vi "RT_MAIN.vi"() -> ()   [LabVIEW 2019]
uses:
  <vilib>/Platform/TimedLoop/XDataNode/timing_clust.ctl
  <vilib>/Platform/TimedLoop/XDataNode/nitl_modes.ctl
  <vilib>/Platform/TimedLoop/XDataNode/wakeup.ctl
  <vilib>/FPGAPlugInAG/cRIO-9040/niLvFpga_Open_cRIO-9040.vi
  <vilib>/rvi/interface/common/dynamic/niFpgaDynamicAddResources.vi
  <vilib>/FPGAPlugInAG/Dynamic/niLvFpga_Reset_Dynamic.vi
  <vilib>/FPGAPlugInAG/Dynamic/niLvFpga_Run_Dynamic.vi
  <vilib>/Utility/error.llb/Error Cluster From Error Code.vi
  <vilib>/rvi/errors/niLvFpgaAdjustHostInterfaceError.vi
  <vilib>/FPGAPlugInAG/Dynamic/niLvFpga_Abort_Dynamic.vi
  <vilib>/FPGAPlugInAG/Dynamic/niLvFpga_Close_Dynamic.vi
  <vilib>/rvi/interface/nirviOpenFPGA/nirviOpenFPGA.xnode
  FPGA Bitfiles/groundtruthproj_FPGATarget_FPGAMAIN_IKH4XQWN-oQ.lvbitx
  FPGA/FPGA_MAIN.vi
  <vilib>/rvi/interface/nirviMethod/nirviMethod.xnode
  <vilib>/Platform/TimedLoop/XDataNode/XDataNode.xnode
  <vilib>/rvi/interface/nirviReadWriteControl/nirviReadWriteControl.xnode
  <vilib>/rvi/interface/nirviCloseFPGA/nirviCloseFPGA.xnode
  <vilib>/Platform/TimedLoop/XDataNode/XDNodeRunTimeDep.lvlib
  <vilib>/NI_Real-Time Target Support.lvlib
  NiFpgaLv.dll
  <vilib>/rvi/interface/Simulation/niFpgaSimulationCallBeginRW.vi
panel:
  out "CPU loads[1].Total (%)":dbl
  out "CPU loads[0].Total (%)":dbl
  out "Saveindex":i32
  out "웨이브폼 차트":T1(graph)
  out "Data 2":sgl[](array[numeric])
  in  "정지":bool
  in  "SAVE":bool
  out "D0 2":bool
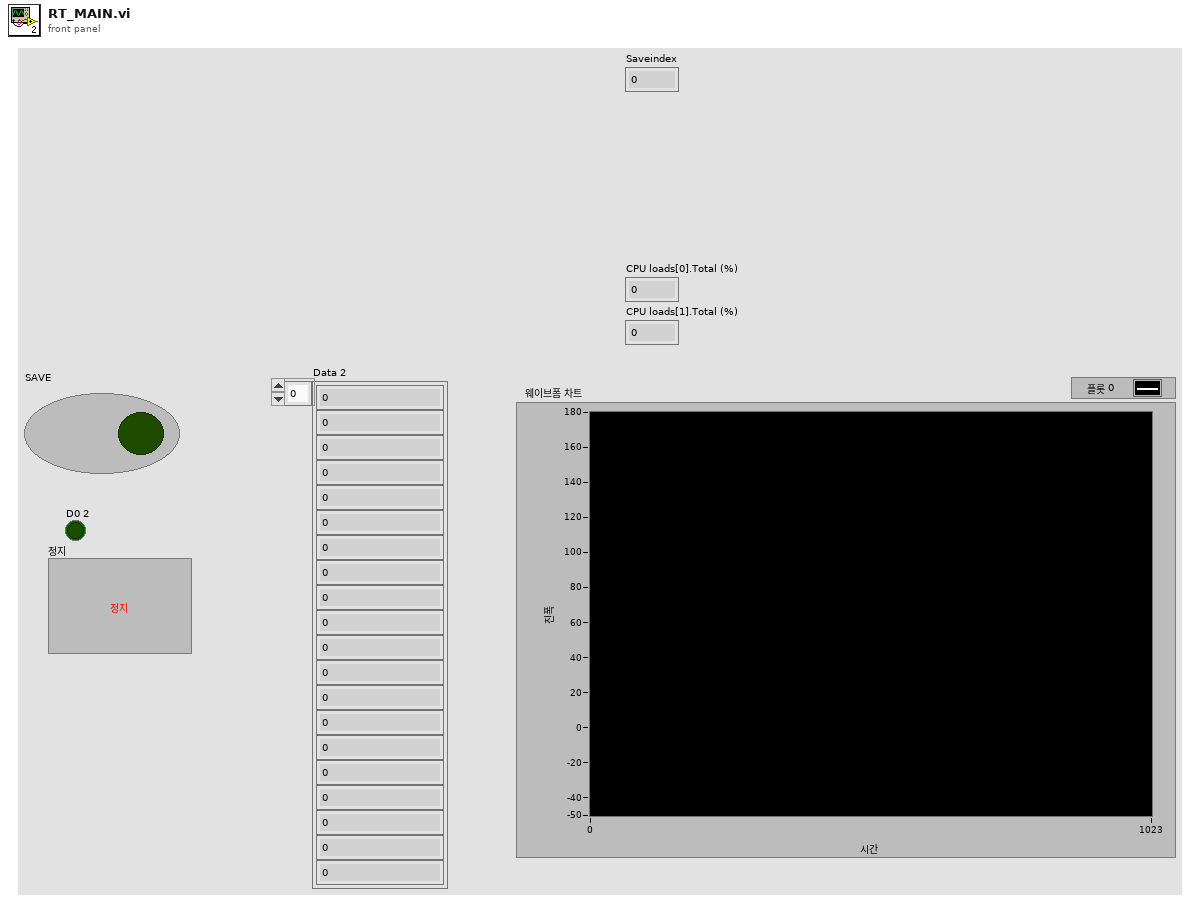
[diagram p1: front panel]
types:
  T1 = cluster{"Data 2[0]":sgl, "Data 2[1]":sgl, "Data 2[2]":sgl, "Data 2[3]":sgl, "Data 2[4]":sgl, "Data 2[5]":sgl, "Data 2[6]":sgl, "Data 2[7]":sgl, "Data 2[8]":sgl, "Data 2[9]":sgl, "Data 2[10]":sgl, "Data 2[11]":sgl, "Data 2[12]":sgl, "Data 2[13]":sgl, "Data 2[14]":sgl, "Data 2[15]":sgl, "Data 2[16]":sgl, "Data 2[17]":sgl, "Data 2[18]":sgl, "Data 2[19]":sgl}
  T2 = cluster{"FPGA_Data":sgl[], "D0":bool, "D1":bool, "cheak":i32, "Loop time":dbl, "Integtrate time":dbl}
  T3 = cluster{"FPGA_Data":sgl[], "Save":bool, "D1":bool, "cheak":i32, "Loop time":dbl, "Integtrate time":dbl}
  T4 = typedef "XDNodeRunTimeDep.lvlib/timing_clust.ctl" = cluster{"Expected End [f-1]":u64, "Actual End [f-1]":u64, "Finished Late? [f-1]":bool, "Expected End [i-1]":u64, "Actual End [i-1]":u64, "Finished Late? [i-1]":bool, "Expected Start [i]":u64, "Actual Start [i]":u64, "Expected Start [f]":u64, "Actual Start [f]":u64, "Source Name":string, "Structure Name":string, "Period":i64, "Deadline":i64, "Offset":i64, "Start":i64, "Priority":i32, "Timeout":i32, "Mode":T5, "Wakeup Reason":T6, "Error":errorcluster, "Source Type":string, "Secondary Source Type":string, "Global End Time":u64, "Global Start Time":u64, "Frame Duration":u64, "Iteration Duration":u64, "Assigned CPU":i32, "I/O Scan Engine Mode":u32}
  T5 = typedef "XDNodeRunTimeDep.lvlib/nitl_modes.ctl" = enum32{"No Change", "Process missed periods, maintain original phase", "Discard missed periods, maintain original phase", "Process missed periods, ignore original phase", "Discard missed periods, ignore original phase"}
  T6 = typedef "XDNodeRunTimeDep.lvlib/wakeup.ctl" = enum32{"Normal", "Aborted", "Asynchronous wakeup", "Timing source error", "Timed loop error", "Timeout"}
  T7 = enum16{"open", "replace", "create", "open or create", "replace or create", "replace or create with confirmation"}
  T8 = cluster{"FPGA_Data":sgl[], "Save":bool, "D1":bool, "cheak":i32, "Loop time":dbl, "Integtrate time":dbl}[]
  T9 = cluster{"IMUS[0]":sgl, "IMUS[1]":sgl, "IMUS[2]":sgl, "IMUS[3]":sgl, "IMUS[4]":sgl, "IMUS[5]":sgl, "IMUS[6]":sgl, "IMUS[7]":sgl, "IMUS[8]":sgl, "IMUS[9]":sgl, "IMUS[10]":sgl, "IMUS[11]":sgl, "IMUS[12]":sgl, "IMUS[13]":sgl, "IMUS[14]":sgl, "IMUS[15]":sgl, "IMUS[16]":sgl, "IMUS[17]":sgl, "IMUS[18]":sgl, "IMUS[19]":sgl}
  T10 = typedef "NI_Real-Time Target Support.lvlib/RT CPU Load.ctl" = cluster{"Total (%)":dbl, "Time Critical (%)":dbl, "Timed Structures (%)":dbl, "High (%)":dbl, "Above Normal (%)":dbl, "Normal (%)":dbl, "Background (%)":dbl, "Idle (%)":dbl, "ISR (%)":dbl}
  T11 = cluster{"CPU loads[0]":T10, "CPU loads[1]":T10, "CPU loads[2]":T10, "CPU loads[3]":T10, "CPU loads[4]":T10, "CPU loads[5]":T10, "CPU loads[6]":T10, "CPU loads[7]":T10, "CPU loads[8]":T10}
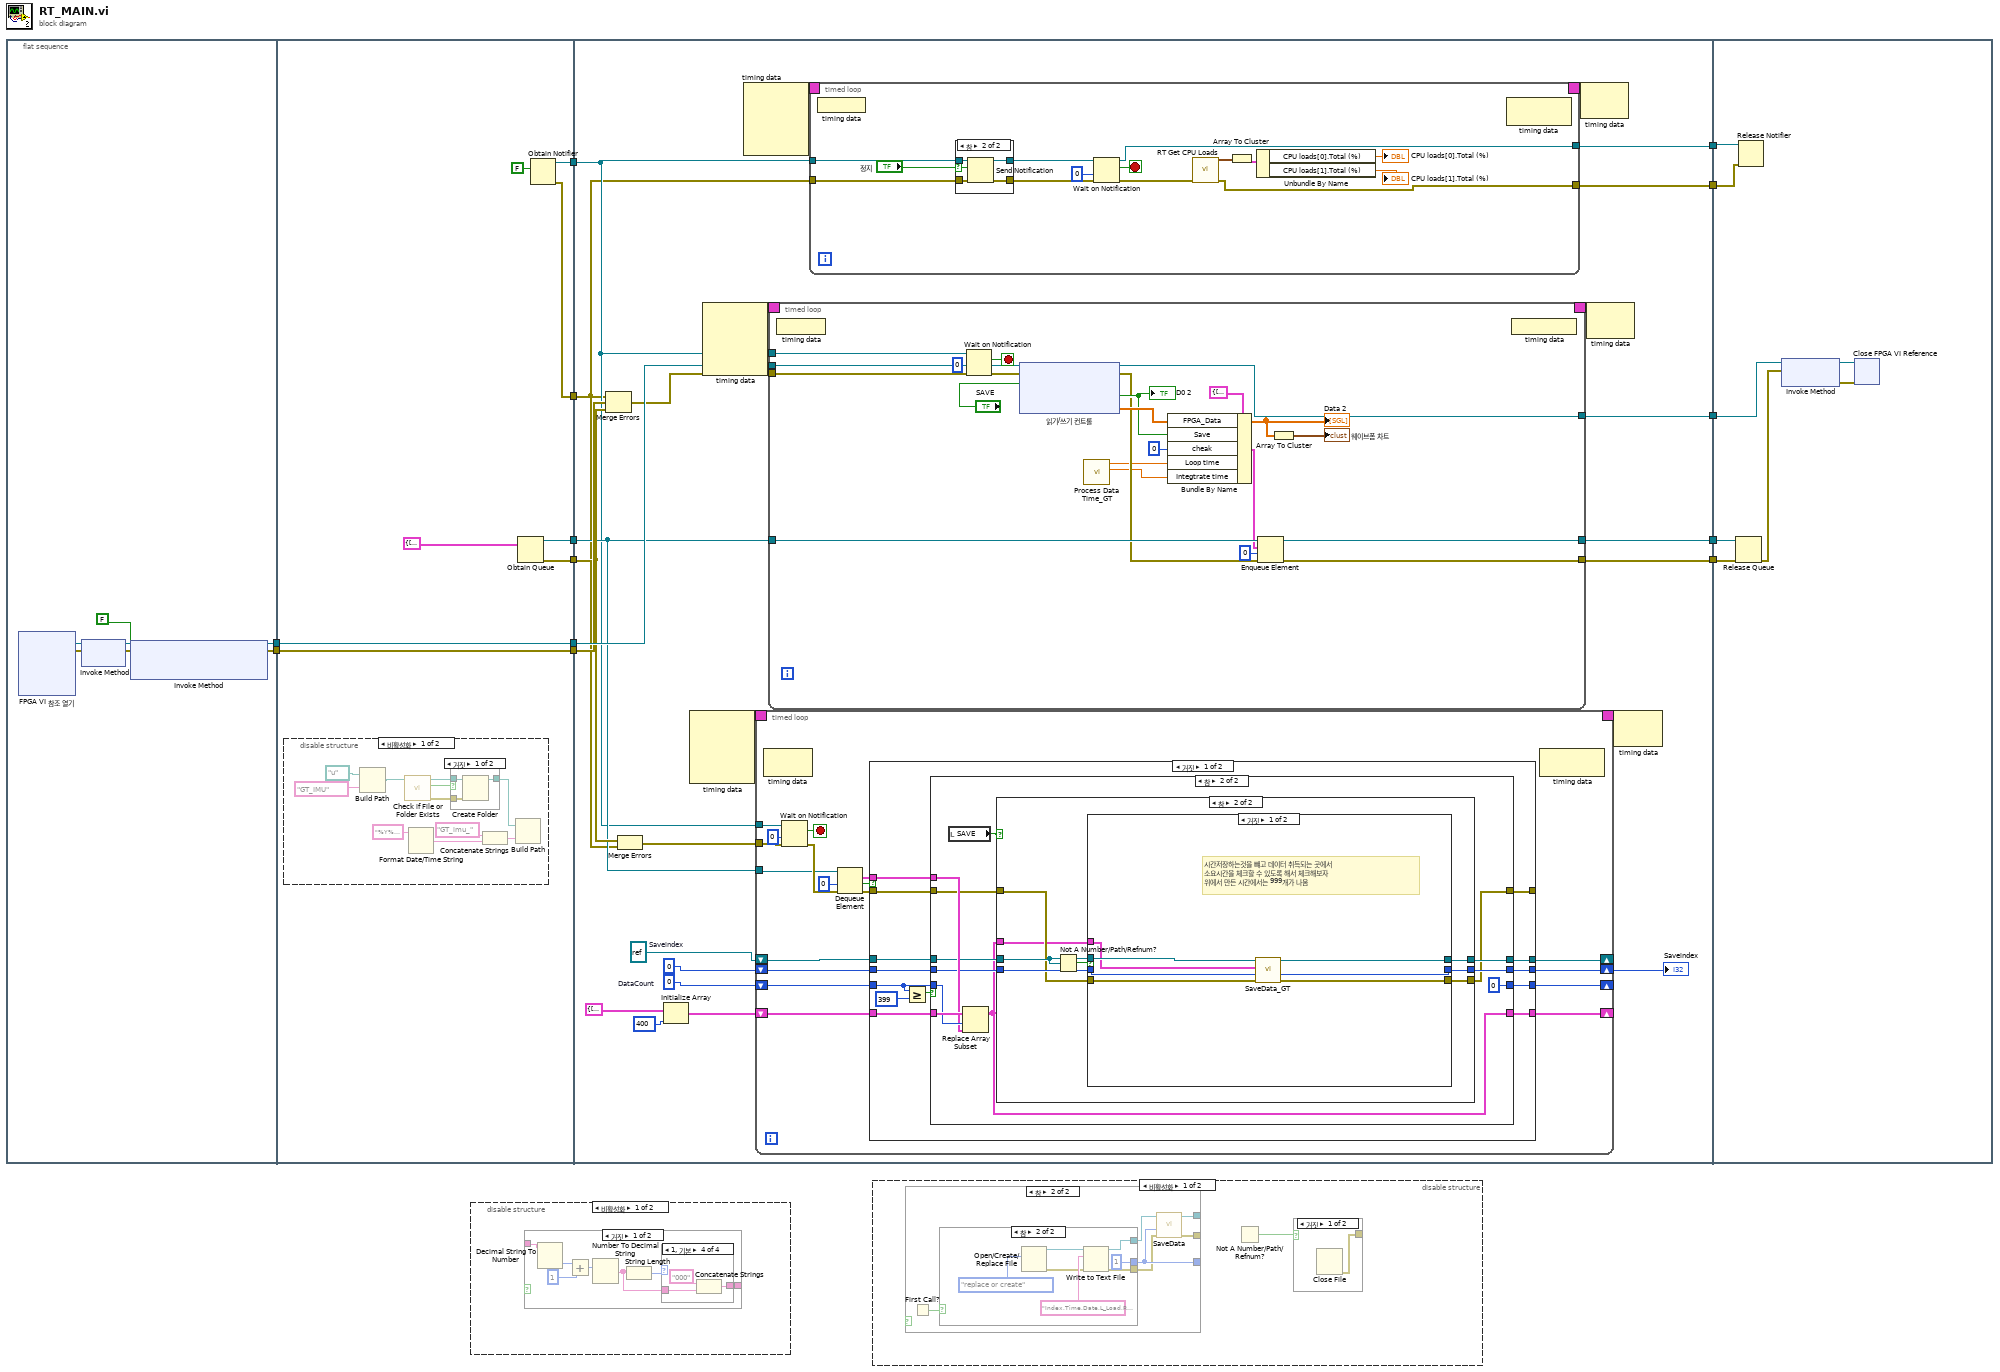
[diagram p0: block diagram]
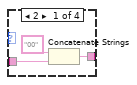
[diagram p2: hidden frame]
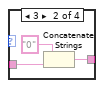
[diagram p3: hidden frame]
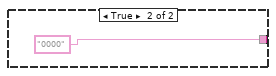
[diagram p5: hidden frame]
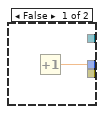
[diagram p9: hidden frame]
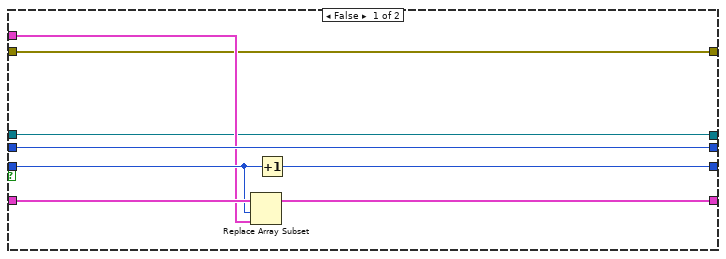
[diagram p14: hidden frame]
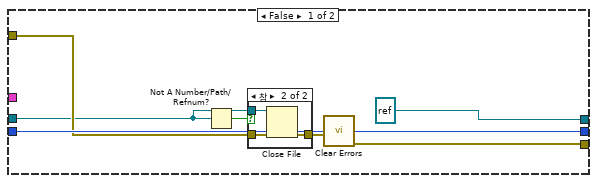
[diagram p15: hidden frame]
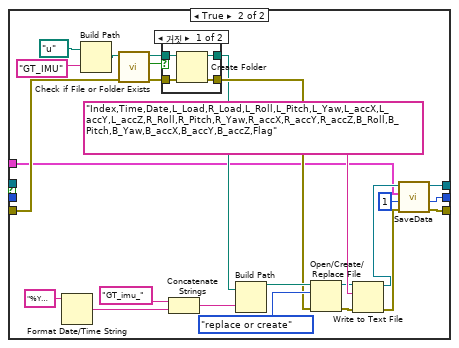
[diagram p17: hidden frame]
diagram:
  n1 = flat-sequence {
    tunnel: [w18] -> w13
    tunnel: [w17] -> w11
    tunnel: w13 -> [w28]
    tunnel: [w28] -> w12
    tunnel: w11 -> [w27]
    tunnel: [w27] -> w10
    tunnel: [w26] -> w8
    tunnel: [w25] -> w7
    tunnel: [w24] -> w4
    tunnel: [w23] -> w3
    tunnel: w12 -> [w67]
    tunnel: w10 -> [w61]
    tunnel: [w66] -> w9
    tunnel: w8 -> [w57]
    tunnel: w7 -> [w59]
    tunnel: [w63] -> w6
    tunnel: [w62] -> w5
    tunnel: w4 -> [w47]
    tunnel: w3 -> [w48]
    tunnel: [w46] -> w2
    tunnel: [w45] -> w1
    tunnel: w9 -> [w242]
    tunnel: w6 -> [w241]
    tunnel: w5 -> [w240]
    tunnel: w2 -> [w238]
    tunnel: w1 -> [w237]
    frame #0 {
      n2 = xnode "FPGA VI 참조 열기"() -> ("FPGA VI 참조 출력"=w16:refnum<k20>, "에러 출력"=w15:errorcluster)  [unwired: 2 in]
      n3 = xnode "Invoke Method"("FPGA VI 참조 입력"=w16, "에러 입력"=w15) -> ("FPGA VI 참조 출력"=w20:refnum<k20>, "에러 출력"=w19:errorcluster)
      n4 = xnode "Invoke Method"("FPGA VI 참조 입력"=w20, "에러 입력"=w19, "완료될 때까지 기다림(거짓)"=FALSE) -> ("FPGA VI 참조 출력"=w18:refnum<k20>, "에러 출력"=w17:errorcluster)
    }
    frame #1 {
      n5 = disable-structure shown="비활성화" {
        frame Disabled {
          n6 = Build Path(base path=path "u:/" ("베이스 경로"), name or relative path="GT_IMU" ("시간 포맷 문자열 (%c)")) -> (appended path=w30:path)
          n7 = call <vilib>:"Check if File or Folder Exists.vi"("path"=w30) -> ("error out"=w29:errorcluster, "file or folder exists?"=w36:bool, "dup path"=w37:path)  [unwired: 8 in]
          n8 = Format Date/Time String(time format string (%c)="%Y%m%d_%H%M%S.csv" ("시간 포맷 문자열 (%c)")) -> (date/time string=w34:string)  [unwired: 2 in]
          n9 = case shown="거짓" w36 {
            tunnel: w37 -> [w42 w43]
            tunnel: [w41 w43] -> w33
            tunnel: w29 -> [w40 _]
            frame False {
              n10 = Create Folder(path (use dialog)=w42, error in=w40) -> (created path=w41:path)  [unwired: 1 in, 2 out]
            }
            frame True {
            }
          }
          n11 = Concatenate Strings("GT_imu_" ("문자열"), w34) -> (w35:string)
          n12 = Build Path(base path=w33, name or relative path=w35) -> ()  [unwired: 1 out]
        }
        frame Enabled {
        }
      }
      n13 = Obtain Queue(element data type=T2 {"FPGA_Data"=[], "D0"=FALSE, "D1"=FALSE, "cheak"=0, "Loop time"=0.0, "Integtrate time"=0.0}) -> (queue out=w26:refnum<queue>, error out=w25:errorcluster)  [unwired: 4 in, 1 out]
      n14 = Obtain Notifier(notification data type=FALSE) -> (notifier out=w23:refnum<notifier>, error out=w24:errorcluster)  [unwired: 3 in, 1 out]
    }
    frame #2 {
      w53 = 0  # DataCount
      w52 = 0  # Saveindex
      n15 = Merge Errors(w47, w61, w59) -> (w60:errorcluster)
      n16 = Merge Errors(w59, w47) -> (w58:errorcluster)
      n17 = Initialize Array(T3 {"FPGA_Data"=[], "Save"=FALSE, "D1"=FALSE, "cheak"=0, "Loop time"=0.0, "Integtrate time"=0.0}, 400 ("차원 크기")) -> (w54:T8)
      n18 = node-c288() -> (w65:T4)  [unwired: 4 in]
      n19 = node-c288() -> (w69:T4)  [unwired: 4 in]
      n20 = node-c288() -> (w50:T4)  [unwired: 4 in]
      n21 = timed-loop {
        timing: w65 -> [_]
        timing-out: [_] -> w64
        tunnel: w58 -> [w112]
        tunnel: w48 -> [w111]
        tunnel: w57 -> [w107]
        shift-right: [w100] -> w51
        shift-left: w52 -> [w103]
        shift-right: [w101] -> _
        shift-left: w53 -> [w104]
        shift-right: [w98] -> _
        shift-left: w54 -> [w102]
        shift-right: [w97] -> _
        shift-left: refnum<file> refnum ("참조 번호") -> [w96]
        stop <- w109 stop-if-true
        n22 = node-c288() -> ()  [unwired: 1 in, 1 out]
        n23 = Wait on Notification(notifier=w111, timeout in ms (-1)=0 ("타임아웃(ms) (-1)"), error in (no error)=w112) -> (notification=w109:bool, error out=w108:errorcluster)  [unwired: 1 in, 2 out]
        n24 = Dequeue Element(queue=w107, timeout in ms (-1)=0 ("타임아웃(ms) (-1)"), error in (no error)=w108) -> (element=w99:T2, timed out?=w106:bool, error out=w105:errorcluster)  [unwired: 1 out]
        n25 = case shown="거짓" w106 {
          tunnel: w105 -> [w122 w206]
          tunnel: w104 -> [w120 w204]
          tunnel: w103 -> [w123 w205]
          tunnel: w102 -> [w121 w203]
          tunnel: [w119 w204] -> w101
          tunnel: [w118 w205] -> w100
          tunnel: w99 -> [w117 _]
          tunnel: [w116 w206] -> _
          tunnel: [w115 w203] -> w98
          tunnel: [w114 w207] -> w97
          tunnel: w96 -> [w113 w207]
          frame False {
            n26 = Greater Or Equal?(x=w120, y=399) -> (x >= y?=w124:bool)
            n27 = case shown="참" w124 {
              tunnel: w123 -> [w130 w141]
              tunnel: w122 -> [w128 w139]
              tunnel: w121 -> [w133 w145]
              tunnel: w120 -> [w132 w144]
              tunnel: [w131 0] -> w119
              tunnel: [w130 w140] -> w118
              tunnel: w117 -> [w129 w143]
              tunnel: [w128 w136] -> w116
              tunnel: [w127 w135] -> w115
              tunnel: [w126 w138] -> w114
              tunnel: w113 -> [w126 w137]
              frame False {
                n28 = Replace Array Subset(array=w133, new element=w129, index=w132) -> (w127:T8)
                n29 = Increment(x=w132) -> (x+1=w131:i32)
              }
              frame True {
                n30 = local read "SAVE"() -> (w134:bool)
                n31 = Replace Array Subset(array=w145, new element=w143, index=w144) -> (w135:T8)
                n32 = case shown="참" w134 {
                  tunnel: w141 -> [w151 w162]
                  tunnel: [w151 w157] -> w140
                  tunnel: w139 -> [w150 w161]
                  tunnel: [refnum<file> refnum ("참조 번호") w159] -> w138
                  tunnel: w137 -> [w148 w163]
                  tunnel: w135 -> [_ w160]
                  tunnel: [w146 w158] -> w136
                  frame False {
                    n33 = Not A Number/Path/Refnum?(number/path/refnum=w148) -> (NaN/Path/Refnum?=w147:bool)
                    n34 = case shown="참" w147 {
                      tunnel: [w153 w156] -> w152
                      tunnel: w150 -> [w153 w155]
                      tunnel: w148 -> [_ w154]
                      frame False {
                      }
                      frame True {
                        n35 = Close File(refnum=w154, error in=w155) -> (error out=w156:errorcluster)  [unwired: 1 out]
                      }
                    }
                    n36 = call <vilib>:"Clear Errors.vi"("error in (no error)"=w152) -> ("error out"=w146:errorcluster)  [unwired: 5 in, 1 out]
                  }
                  frame True {
                    n37 = Not A Number/Path/Refnum?(number/path/refnum=w163) -> (NaN/Path/Refnum?=w164:bool)
                    n38 = case shown="거짓" w164 {
                      tunnel: w163 -> [w171 _]
                      tunnel: w162 -> [w169 _]
                      tunnel: w161 -> [w168 w186]
                      tunnel: w160 -> [w170 w172]
                      tunnel: [w165 w182] -> w159
                      tunnel: [w167 w180] -> w158
                      tunnel: [w166 w181] -> w157
                      frame False {
                        # "시간저장하는것을 뺴고 데이터 취득되는 곳에서 \n소요시간을 체크할 수 있도록 해서 체크해보자\n위에서 만든 시간에서는 999개가 나옴"
                        n39 = call "SaveData_GT.vi"("에러 입력"=w168, "Index"=w169, "배열"=w170, "참조번호"=w171) -> ("에러 출력"=w167:errorcluster, "Index 2"=w166:i32, "참조 번호 출력"=w165:refnum<file>)  [unwired: 5 in]
                      }
                      frame True {
                        n40 = Format Date/Time String(time format string (%c)="%Y%m%d_%H%M%S.csv" ("시간 포맷 문자열 (%c)")) -> (date/time string=w191:string)  [unwired: 2 in]
                        n41 = Build Path(base path=path "u:/" ("베이스 경로"), name or relative path="GT_IMU" ("시간 포맷 문자열 (%c)")) -> (appended path=w188:path)
                        n42 = call <vilib>:"Check if File or Folder Exists.vi"("error in (no error)"=w186, "path"=w188) -> ("error out"=w187:errorcluster, "file or folder exists?"=w193:bool, "dup path"=w194:path)  [unwired: 7 in]
                        n43 = case shown="거짓" w193 {
                          tunnel: w194 -> [w200 w202]
                          tunnel: [w199 w202] -> w175
                          tunnel: w187 -> [w198 w201]
                          tunnel: [w197 w201] -> w176
                          frame False {
                            n44 = Create Folder(path (use dialog)=w200, error in=w198) -> (created path=w199:path, error out=w197:errorcluster)  [unwired: 1 in, 1 out]
                          }
                          frame True {
                          }
                        }
                        n45 = Concatenate Strings("GT_imu_" ("문자열"), w191) -> (w192:string)
                        n46 = Build Path(base path=w175, name or relative path=w192) -> (appended path=w179:path)
                        n47 = Open/Create/Replace File(file path (use dialog)=w179, error in=w176, operation (0:open)=T7."replace or create" ("동작(0:open)")) -> (refnum out=w174:refnum<file>, error out=w184:errorcluster)  [unwired: 3 in, 1 out]
                        n48 = Write to Text File(file (use dialog)=w174, text="Index,Time,Date,L_Load,R_Load,L_Roll,L_Pitch,L_Yaw,L_accX,L_accY,L_accZ,R_Roll,R_Pitch,R_Yaw,R_accX,R_accY,R_accZ,B_Roll,B_Pitch,B_Yaw,B_accX,B_accY,B_accZ,Flag" ("텍스트"), error in=w184) -> (refnum out=w173:refnum<file>, error out=w177:errorcluster)  [unwired: 1 in, 1 out]
                        n49 = call "SaveData.vi"("에러 입력"=w177, "Index"=1, "배열"=w172, "참조번호"=w173) -> ("에러 출력"=w180:errorcluster, "Index 2"=w181:i32, "참조 번호 출력"=w182:refnum<file>)  [unwired: 5 in]
                      }
                    }
                  }
                }
              }
            }
          }
          frame True {
          }
        }
        n50 = node-c288() -> ()  [unwired: 1 in, 1 out]
      }
      "Saveindex" <- w51
      n51 = timed-loop {
        timing: w69 -> [_]
        timing-out: [_] -> w68
        tunnel: w67 -> [w232]
        tunnel: [w231] -> w66
        tunnel: w57 -> [w227]
        tunnel: [w224] -> w63
        tunnel: [w223] -> w62
        tunnel: w60 -> [w215]
        tunnel: w48 -> [w216]
        stop <- w220 stop-if-true
        n52 = node-c288() -> ()  [unwired: 1 in]
        n53 = Wait on Notification(notifier=w216, timeout in ms (-1)=0 ("타임아웃(ms) (-1)"), error in (no error)=w215) -> (notification=w220:bool, error out=w221:errorcluster)  [unwired: 1 in, 2 out]
        n54 = xnode "읽기/쓰기 컨트롤"("FPGA VI 참조 입력"=w232, "에러 입력"=w221, "Save_que"="SAVE") -> ("FPGA VI 참조 출력"=w231:refnum<k20>, "에러 출력"=w222:errorcluster, "Save_que_indicator"=w228:bool, "IMUS"=w229:sgl[])
        "D0 2" <- w228
        "Data 2" <- w229
        n55 = call "Process Data Time_GT.vi"() -> ("Integrate time"=w213:dbl, "Loop time"=w214:dbl)  [unwired: 10 in]
        n56 = Bundle By Name(cluster=T3 {"FPGA_Data"=[], "Save"=FALSE, "D1"=FALSE, "cheak"=0, "Loop time"=0.0, "Integtrate time"=0.0}, "FPGA_Data"=w229, "Save"=w228, "cheak"=0, "Loop time"=w214, "Integtrate time"=w213) -> (w226:T3)
        n57 = Enqueue Element(queue=w227, element=w226, timeout in ms (-1)=0 ("타임아웃(ms) (-1)"), error in (no error)=w222) -> (queue out=w224:refnum<queue>, error out=w223:errorcluster)  [unwired: 1 out]
        n58 = Array To Cluster(array=w229) -> (cluster=→"웨이브폼 차트":T9)
        n59 = node-c288() -> ()  [unwired: 1 out]
      }
      n60 = timed-loop {
        timing: w50 -> [_]
        timing-out: [_] -> w49
        tunnel: w48 -> [w82]
        tunnel: w47 -> [w81]
        tunnel: [w71] -> w45
        tunnel: [w70] -> w46
        stop <- w77 stop-if-true
        n61 = node-c288() -> ()  [unwired: 1 in]
        n62 = case shown="참" "정지" {
          selector: "정지" -> [_ w86]
          tunnel: w82 -> [w85 w90]
          tunnel: w81 -> [w84 w89]
          tunnel: [w84 w88] -> w78
          tunnel: [w85 w87] -> w79
          frame False {
          }
          frame True {
            n63 = Send Notification(notification=w86, notifier=w90, error in (no error)=w89) -> (notifier out=w87:refnum<notifier>, error out=w88:errorcluster)
          }
        }
        n64 = Wait on Notification(notifier=w79, timeout in ms (-1)=0 ("타임아웃(ms) (-1)"), error in (no error)=w78) -> (notifier out=w70:refnum<notifier>, notification=w77:bool, error out=w76:errorcluster)  [unwired: 1 in, 1 out]
        n65 = call <vilib>:"RT Get CPU Loads.vi"("error in (no error)"=w76) -> ("error out"=w71:errorcluster, "CPU loads"=w75:T10[])  [unwired: 9 in]
        n66 = Array To Cluster(array=w75) -> (cluster=w74:T11)
        n67 = Unbundle By Name(w74) -> ("CPU loads[0].Total (%)"=→"CPU loads[0].Total (%)":dbl, "CPU loads[1].Total (%)"=→"CPU loads[1].Total (%)":dbl)
        n68 = node-c288() -> ()  [unwired: 1 in, 1 out]
      }
      n69 = node-c288(w49) -> ()  [unwired: 1 out]
      n70 = node-c288(w68) -> ()  [unwired: 1 out]
      n71 = node-c288(w64) -> ()  [unwired: 1 out]
    }
    frame #3 {
      n72 = Release Queue(queue=w241, error in (no error)=w240) -> (error out=w239:errorcluster)  [unwired: 1 in, 2 out]
      n73 = Release Notifier(notifier=w238, error in (no error)=w237) -> ()  [unwired: 1 in, 3 out]
      n74 = xnode "Invoke Method"("FPGA VI 참조 입력"=w242, "에러 입력"=w239) -> ("FPGA VI 참조 출력"=w244:refnum<k20>, "에러 출력"=w243:errorcluster)
      n75 = xnode "Close FPGA VI Reference"("FPGA VI 참조 입력"=w244, "에러 입력"=w243) -> ()  [unwired: 1 out]
    }
  }
  n76 = disable-structure shown="비활성화" {
    frame Disabled {
      n77 = case shown="거짓" {
        selector: _ -> [_ _]
        tunnel: _ -> [w251 _]
        tunnel: [w245 "0000"] -> _
        frame False {
          n78 = Decimal String To Number(string=w251) -> (number=w250:i32)  [unwired: 2 in, 1 out]
          n79 = Add(x=w250, y=1) -> (x+y=w248:i32)
          n80 = Number To Decimal String(number=w248) -> (decimal integer string=w246:string)  [unwired: 1 in]
          n81 = String Length(string=w246) -> (length=w247:i32)
          n82 = case shown="1, 기본" w247 {
            tunnel: w246 -> [w253 w256 w258 w261]
            tunnel: [w252 w255 w258 w259] -> w245
            frame 2 {
              n83 = Concatenate Strings("00" ("문자열"), w253) -> (w252:string)
            }
            frame 3 {
              n84 = Concatenate Strings("0" ("문자열"), w256) -> (w255:string)
            }
            frame 4 {
            }
            frame 1, Default {
              n85 = Concatenate Strings("000" ("문자열"), w261) -> (w259:string)
            }
          }
        }
        frame True {
        }
      }
    }
    frame Enabled {
    }
  }
  n86 = disable-structure shown="비활성화" {
    frame Disabled {
      n87 = case shown="참" {
        selector: _ -> [_ _]
        tunnel: [_ w270] -> _
        tunnel: [_ w269] -> _
        tunnel: [_ w267] -> _
        frame False {
        }
        frame True {
          n88 = First Call?() -> (First Call?: T/F=w268:bool)
          n89 = case shown="참" w268 {
            tunnel: [w271 1 ("Index")] -> w267
            tunnel: [_ w277] -> w266
            tunnel: [_ w276] -> w265
            frame False {
              n90 = Increment() -> (x+1=w271:dbl)  [unwired: 1 in]
            }
            frame True {
              n91 = Open/Create/Replace File(operation (0:open)=T7."replace or create" ("동작(0:open)")) -> (refnum out=w273:refnum<file>, error out=w274:errorcluster)  [unwired: 5 in, 1 out]
              n92 = Write to Text File(file (use dialog)=w273, text="Index,Time,Date,L_Load,R_Load,L_Roll,L_Pitch,L_Yaw,L_accX,L_accY,L_accZ,R_Roll,R_Pitch,R_Yaw,R_accX,R_accY,R_accZ,B_Roll,B_Pitch,B_Yaw,B_accX,B_accY,B_accZ,Flag" ("텍스트"), error in=w274) -> (refnum out=w277:refnum<file>, error out=w276:errorcluster)  [unwired: 1 in, 1 out]
            }
          }
          n93 = call "SaveData.vi"("에러 입력"=w265, "Index"=w267, "참조번호"=w266) -> ("에러 출력"=w269:errorcluster, "참조 번호 출력"=w270:refnum<file>)  [unwired: 6 in, 1 out]
        }
      }
      n94 = Not A Number/Path/Refnum?() -> (NaN/Path/Refnum?=w263:bool)  [unwired: 1 in]
      n95 = case shown="거짓" w263 {
        tunnel: [w264 _] -> _
        frame False {
          n96 = Close File() -> (error out=w264:errorcluster)  [unwired: 2 in, 1 out]
        }
        frame True {
        }
      }
    }
    frame Enabled {
    }
  }
